vi "Draw Selected Rectangle.vi"(8 "New Node":T1={"Node Type"=enum."Path", "ID"=0, "Path Data"={"Path Name"="", "Outcome Name"=""}, "Single Cmd Info"={"Name"="", "CPTM.DataType"=variant, "All Control Values Variant"=[], "icon full"={"image type"=0, "image depth"=0, "image"=[], "mask"=[], "colors"=[], "Rectangle"={"left"=0, "top"=0, "right"=0, "bottom"=0}}, "icon scaled"={"image type"=0, "image depth"=0, "image"=[], "mask"=[], "colors"=[], "Rectangle"={"left"=0, "top"=0, "right"=0, "bottom"=0}}, "Path"=path "", "Subsystem Color"=16777216}, "Child ID"=[], "Parent ID"=0, "Drawing Info"={"X"=0, "Y"=0, "Width"=0, "Height"=0}}, 9 "Prev. Node":T1[](array[typedef]), 11 "2D Picture":picture) -> (3 "Decision Tree Out":picture)   [LabVIEW 2025]
uses:
  Types/Sequencing Tree Node.ctl
  Types/Single Cmd Info.ctl
  <vilib>/picture/picture.llb/imagedata.ctl
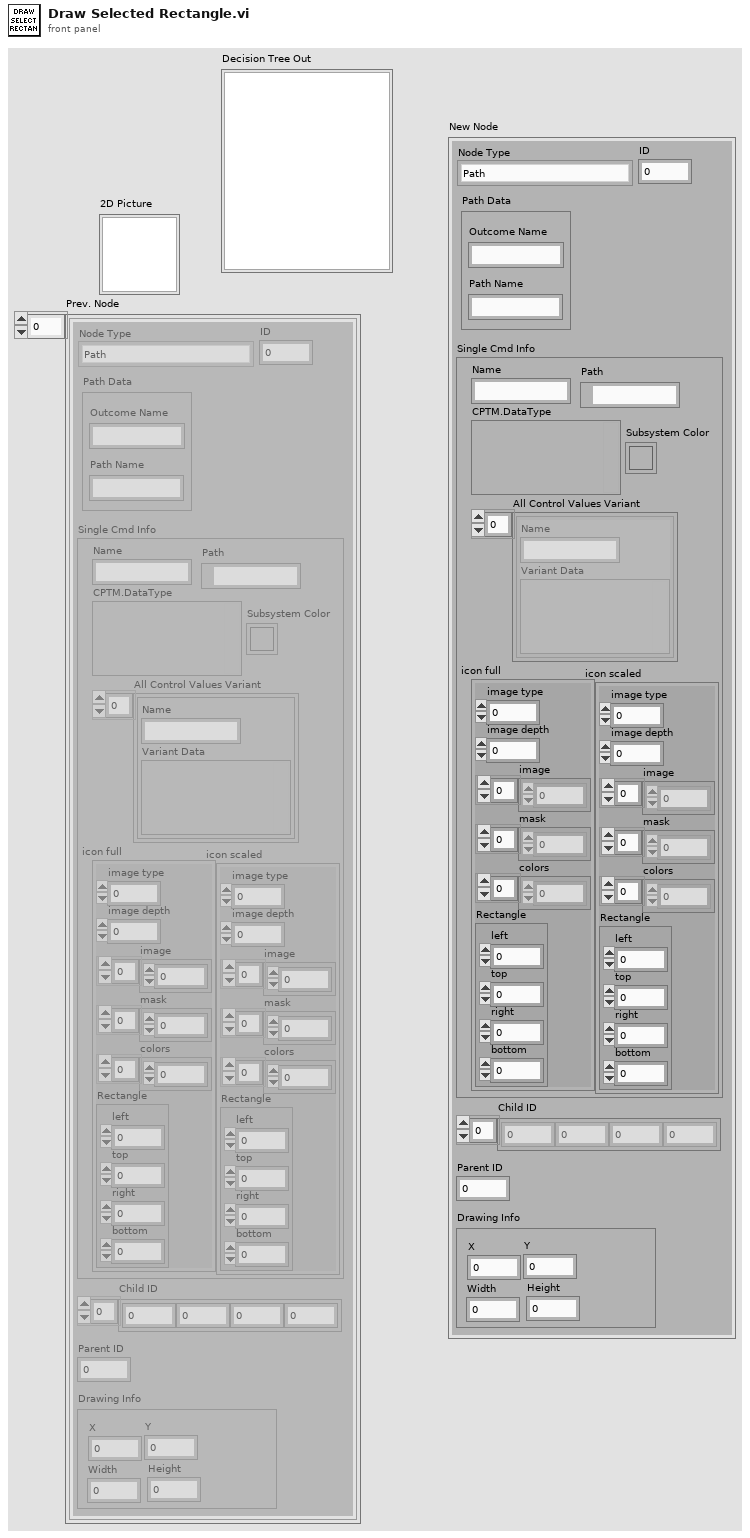
[diagram p1: front panel]
types:
  T1 = typedef "Sequencing Tree Node.ctl" = cluster{"Node Type":enum16{"Path", "Command", "Leaf"}, "ID":i16, "Path Data":cluster{"Path Name":string, "Outcome Name":string}, "Single Cmd Info":T2, "Child ID":i32[], "Parent ID":i32, "Drawing Info":cluster{"X":i32, "Y":i32, "Width":i32, "Height":i32}}
  T2 = typedef "Single Cmd Info.ctl" = cluster{"Name":string, "CPTM.DataType":variant, "All Control Values Variant":cluster{"Name":string, "Variant Data":variant}[], "icon full":T3, "icon scaled":T3, "Path":path, "Subsystem Color":u32}
  T3 = typedef "imagedata.ctl" = cluster{"image type":i32, "image depth":i32, "image":u8[], "mask":u8[], "colors":u32[], "Rectangle":cluster{"left":i16, "top":i16, "right":i16, "bottom":i16}}
  T4 = cluster{"Width":i16, "Style":enum32{"Solid", "Dash", "Dot", "DashDot", "DashDotDot"}}
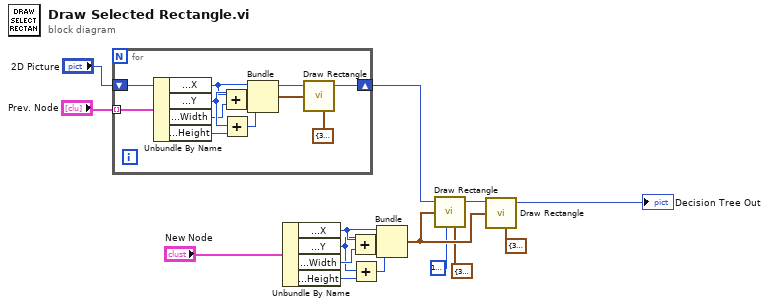
[diagram p0: block diagram]
diagram:
  n1 = for {
    tunnel: "Prev. Node" -> [w21] mode=indexing
    shift-right: [w18] -> w1
    shift-left: "2D Picture" -> [w19]
    n2 = Unbundle By Name(w21) -> ("Drawing Info.X"=w24:i32, "Drawing Info.Y"=w27:i32, "Drawing Info.Width"=w22:i32, "Drawing Info.Height"=w23:i32)
    n3 = Add(x=w24, y=w22) -> (x+y=w25:i32)
    n4 = Add(x=w27, y=w23) -> (x+y=w26:i32)
    n5 = Bundle("X"=w24, "Y"=w27, w25, w26) -> (w20:cluster{"X":i32, "Y":i32, i32, i32})  [unwired: 1 in]
    n6 = call <vilib>:"Draw Rectangle.vi"("picture"=w19, "rect"=w20, "pen"=T4 {"Width"=3, "Style"=enum."Solid"}) -> ("new picture"=w18:picture)  [unwired: 6 in]
  }
  n7 = Unbundle By Name("New Node") -> ("Drawing Info.X"=w11:i32, "Drawing Info.Y"=w8:i32, "Drawing Info.Width"=w13:i32, "Drawing Info.Height"=w12:i32)
  n8 = Add(x=w11, y=w13) -> (x+y=w10:i32)
  n9 = Add(x=w8, y=w12) -> (x+y=w9:i32)
  n10 = Bundle("X"=w11, "Y"=w8, w10, w9) -> (w7:cluster{"X":i32, "Y":i32, i32, i32})  [unwired: 1 in]
  n11 = call <vilib>:"Draw Rectangle.vi"("picture"=w1, "rect"=w7, "color(black)"=u32 16777226, "pen"=T4 {"Width"=3, "Style"=enum."Solid"}) -> ("new picture"=w15:picture)  [unwired: 5 in]
  n12 = call <vilib>:"Draw Rectangle.vi"("picture"=w15, "rect"=w7, "pen"=T4 {"Width"=3, "Style"=enum."Dash"}) -> ("new picture"=→"Decision Tree Out":picture)  [unwired: 6 in]
